vi "Overwrite Live Array.vi"(8 "error in (no error)":errorcluster, 9 "Live Array":T1[](array[typedef]), 10 "Cache Array":T1[](array[typedef])) -> (0 "error out":errorcluster, 3 "Record Array":T1[](array[typedef]))   [LabVIEW 2026, in "Processing_Engine.lvlib"]
uses:
  Processing_Engine.lvlib
  controls/Messaging Payloads/Processed Calibration Point.ctl
  controls/UI/Direction.ctl
  Test Status.ctl
  Settings/Settings.lvlib
  Analysis/Analysis.lvlib
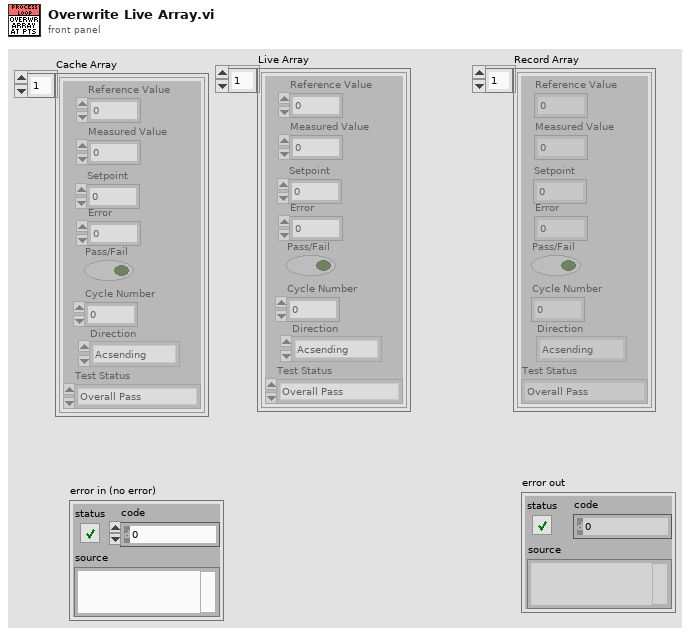
[diagram p1: front panel]
types:
  T1 = typedef "Processed Calibration Point.ctl" = cluster{"Reference Value":dbl, "Measured Value":dbl, "Error":dbl, "Pass/Fail":bool, "Setpoint":dbl, "Cycle Number":i32, "Direction":T2, "Test Status":T3}
  T2 = typedef "Settings.lvlib/Direction.ctl" = enum16{"Acsending", "Descending"}
  T3 = typedef "Analysis.lvlib/Test Status.ctl" = enum16{"Overall Pass", "Overall Fail", "Test Running"}
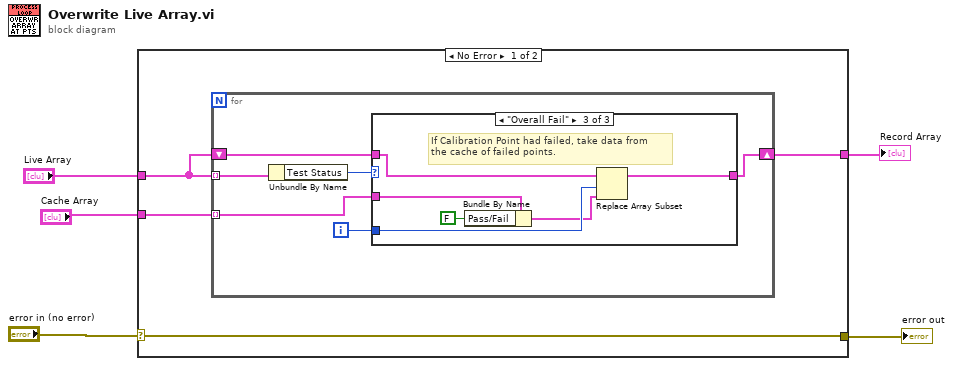
[diagram p0: block diagram]
diagram:
  n1 = case shown="No Error" "error in (no error)" {
    selector: "error in (no error)" -> [w9 w25]
    tunnel: [w9 w25] -> w4
    tunnel: "Live Array" -> [w7 w24]
    tunnel: [w8 w24] -> w1
    tunnel: "Cache Array" -> [w6 _]
    frame No Error {
      n2 = for {
        tunnel: w6 -> [w12] mode=indexing
        tunnel: w7 -> [w13] mode=indexing
        shift-right: [w11] -> w8
        shift-left: w7 -> [w10]
        i -> [w15]
        n3 = Unbundle By Name(w13) -> ("Test Status"=w14:T3)
        n4 = case shown="\"Overall Fail\"" w14 {
          tunnel: w15 -> [_ _ w23]
          tunnel: [w16 w17 w21] -> w11
          tunnel: w12 -> [_ _ w20]
          tunnel: w10 -> [w16 w17 w22]
          frame "Overall Pass" {
            # "If Calibration Point had passed, let recorded \nvalue pass through, as is."
          }
          frame "Test Running" {
          }
          frame "Overall Fail" {
            # "If Calibration Point had failed, take data from \nthe cache of failed points."
            n5 = Bundle By Name(cluster=w20, "Pass/Fail"=FALSE) -> (w18:T1)
            n6 = Replace Array Subset(array=w22, new element=w18, index=w23) -> (w21:T1[])
          }
        }
      }
    }
    frame Error {
    }
  }
  "error out" <- w4
  "Record Array" <- w1
